vi "DiffCompare.vi"(0 "Comparison":T1, 2 "X":dbl, 3 "Y":dbl, 4 "Absolute Diff?":bool, 5 "Threshold":dbl) -> (7 "Result":bool)   [LabVIEW 2012]
uses:
  LiteDifferControl.ctl
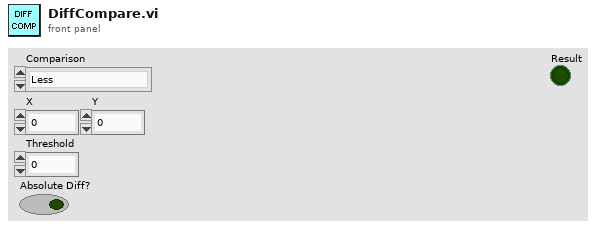
[diagram p1: front panel]
types:
  T1 = typedef "LiteDifferControl.ctl" = enum16{"Less", "Greater"}
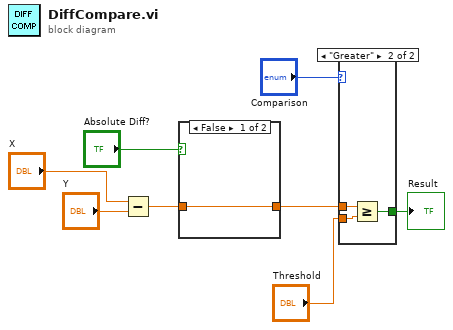
[diagram p0: block diagram]
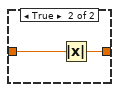
[diagram p2: hidden frame]
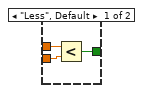
[diagram p3: hidden frame]
diagram:
  n1 = Subtract(x="X", y="Y") -> (x-y=w3:dbl)
  n2 = case shown="False" "Absolute Diff?" {
    tunnel: [w9 w10] -> w5
    tunnel: w3 -> [w9 w11]
    frame False {
    }
    frame True {
      n3 = Absolute Value(x=w11) -> (abs(x)=w10:dbl)
    }
  }
  n4 = case shown="\"Greater\"" "Comparison" {
    tunnel: w5 -> [w14 w17]
    tunnel: "Threshold" -> [w13 w16]
    tunnel: [w12 w15] -> w4
    frame "Less", Default {
      n5 = Less?(x=w14, y=w13) -> (x < y?=w12:bool)
    }
    frame "Greater" {
      n6 = Greater Or Equal?(x=w17, y=w16) -> (x >= y?=w15:bool)
    }
  }
  "Result" <- w4
